vi "Build Dependent Hierarchy Generator Recursive.vi"(0 "Working Set":refnum<data-value>, 5 "Next Root":refnum<data-value>, 11 "error in (no error)":errorcluster) -> (15 "error out":errorcluster)   [LabVIEW 2017, in "CL_G3_VIComponentBuilder.lvlib" / "Build Analyzer.lvclass"]
doc: "The recursive call that enables bubble up analysis."
uses:
  Build Analyzer.lvclass
  <userlib>/_Cirrus Logic/LabVIEW Container/Source/Container/Container.lvclass
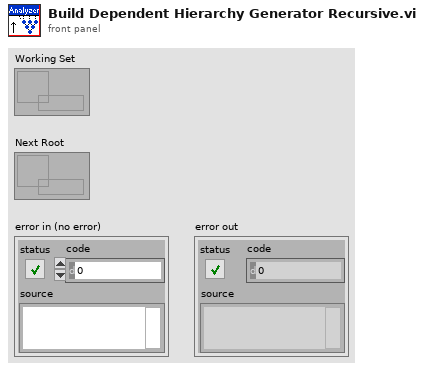
[diagram p1: front panel]
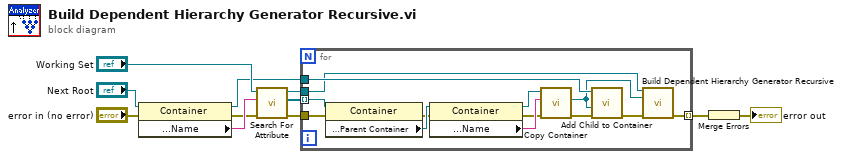
[diagram p0: block diagram]
diagram:
  n1 = property class="Container"(reference="Next Root", error in="error in (no error)") -> (reference out=w5:refnum<data-value>, error out=w2:errorcluster, "Palette VIs:Property Definitions:Name"=w4:string)
  n2 = call <userlib>:"Search For Attribute.vi"("error in (no error)"=w2, "Attribute Name"=w4, "Container"="Working Set") -> ("error out"=w1:errorcluster, "Containers With Attribute"=w7:refnum<data-value>[], "dup Container"=w8:refnum<data-value>)  [unwired: 5 in, 1 out]
  n3 = for {
    tunnel: w8 -> [w20]
    tunnel: [w24] -> w11 mode=indexing
    tunnel: w7 -> [w23] mode=indexing
    tunnel: w5 -> [w21]
    tunnel: w1 -> [w15]
    n4 = property class="Container"(reference=w23, error in=w15) -> (error out=w14:errorcluster, "Palette VIs:Property Definitions:Parent Container"=w18:refnum<data-value>)  [unwired: 1 out]
    n5 = property class="Container"(reference=w18, error in=w14) -> (reference out=w16:refnum<data-value>, error out=w13:errorcluster, "Palette VIs:Property Definitions:Name"=w17:string)
    n6 = call <userlib>:"Copy Container.vi"("error in (no error)"=w13, "New Container Name"=w17, "Container"=w16) -> ("error out"=w12:errorcluster, "New Container"=w19:refnum<data-value>)  [unwired: 6 in, 1 out]
    n7 = call <userlib>:"Add Child to Container.vi"("error in (no error)"=w12, "Child Container"=w19, "Container"=w21) -> ("error out"=w22:errorcluster)  [unwired: 6 in, 2 out]
    n8 = call "Build Dependent Hierarchy Generator Recursive.vi"("Working Set"=w20, "Next Root"=w19, "error in (no error)"=w22) -> ("error out"=w24:errorcluster)  [unwired: 12 in]
  }
  n9 = Merge Errors(w11) -> (→"error out":errorcluster)
